vi "ZeitgrafBehandlung.vi"(6 "MaxArrayGröße":u16, 7 "error in":errorcluster, 8 "Temp-ArrayIn":dbl[](array[numeric]), 9 "Neue Temp":dbl, 10 "Neuer Zeitstempel":timestamp, 11 "Zeitstempel-ArrayIn":timestamp[](array[timestamp])) -> (0 "Temp-ArrayOut":dbl[](array[numeric]), 3 "Zeitstempel-ArrayOut":timestamp[](array[timestamp]), 4 "Temp-ZeitKurve":T1(graph), 5 "error out":errorcluster)   [LabVIEW 2024]
doc: "Dieses VI fügt eine Zeitstempel-Array und ein Werte-Array zusammen um Kurven anzuzeigen\nDabei werden die 2 Arrays zusätzlich verwaltet und auf eine Eingangsgröße beschränkt"
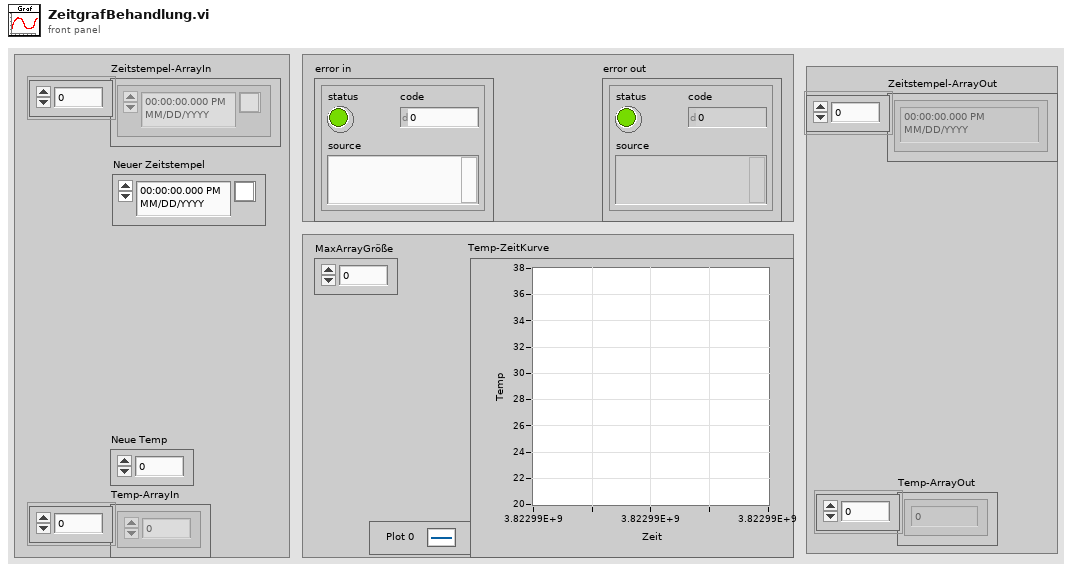
[diagram p1: front panel]
types:
  T1 = cluster{"Zeitstempel-ArrayIn ":timestamp[], "Temp-ArrayIn":dbl[]}
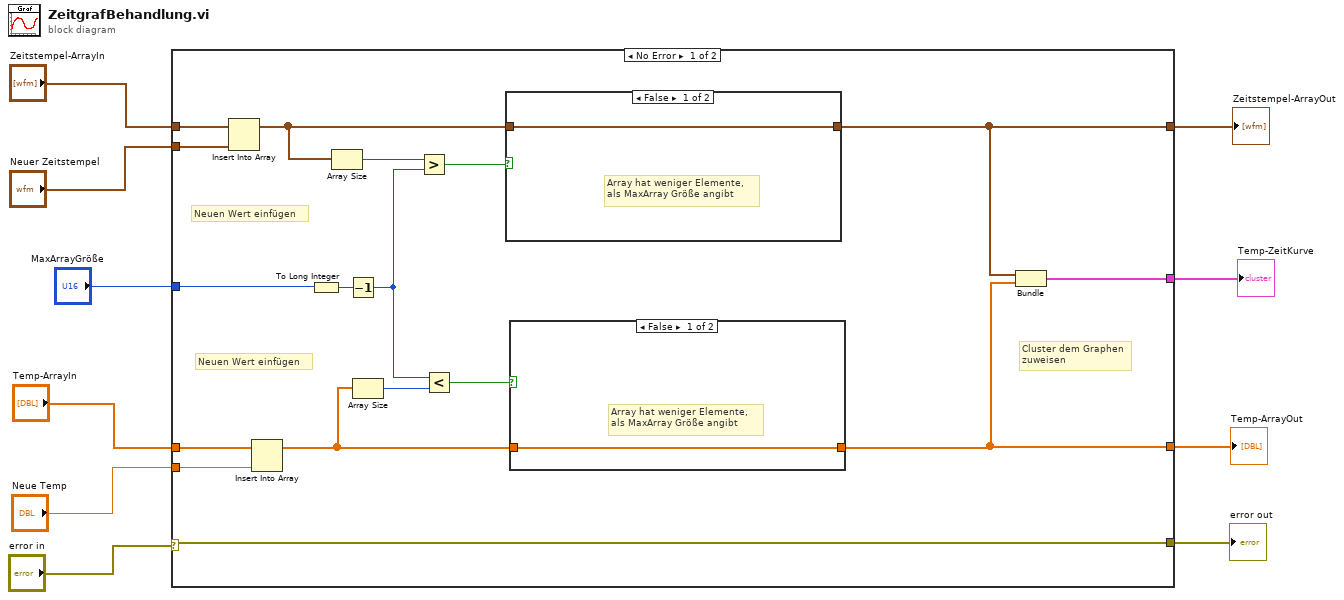
[diagram p0: block diagram]
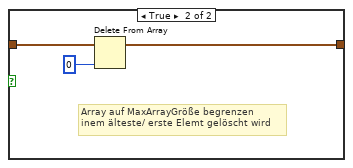
[diagram p2: hidden frame]
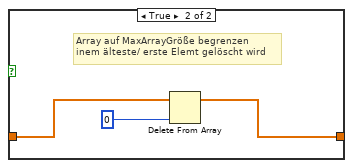
[diagram p3: hidden frame]
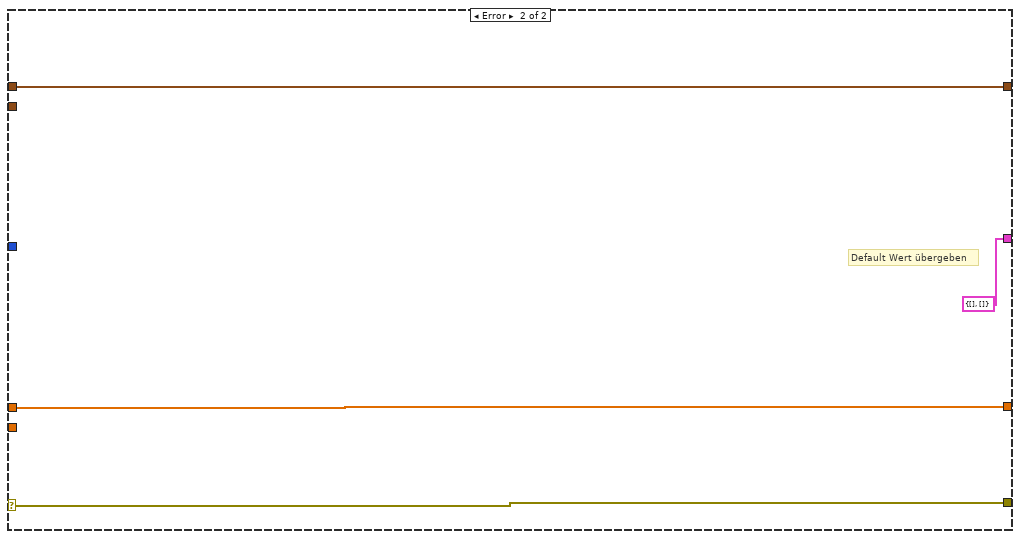
[diagram p4: hidden frame]
diagram:
  n1 = case shown="No Error" "error in" {
    selector: "error in" -> [w27 w38]
    tunnel: [w27 w38] -> w9
    tunnel: "Temp-ArrayIn" -> [w25 w39]
    tunnel: "Neue Temp" -> [w24 _]
    tunnel: "MaxArrayGröße" -> [w23 _]
    tunnel: "Zeitstempel-ArrayIn" -> [w22 w37]
    tunnel: "Neuer Zeitstempel" -> [w21 _]
    tunnel: [w15 w39] -> w3
    tunnel: [w19 T1 {"Zeitstempel-ArrayIn "=[], "Temp-ArrayIn"=[]}] -> w2
    tunnel: [w16 w37] -> w1
    frame No Error {
      # "Neuen Wert einfügen"
      # "Neuen Wert einfügen"
      # "Cluster dem Graphen zuweisen"
      n2 = Insert Into Array(array=w22, new element=w21) -> (w20:timestamp[])  [unwired: 1 in]
      n3 = Insert Into Array(array=w25, new element=w24) -> (w26:dbl[])  [unwired: 1 in]
      n4 = To Long Integer(number=w23) -> (32bit integer=w18:i32)
      n5 = Array Size(array=w20) -> (size(s)=w13:i32)
      n6 = Decrement(x=w18) -> (x-1=w12:i32)
      n7 = Array Size(array=w26) -> (size(s)=w11:i32)
      n8 = Greater?(x=w13, y=w12) -> (0:w14:bool)
      n9 = Less?(x=w12, y=w11) -> (x < y?=w17:bool)
      n10 = case shown="False" w14 {
        tunnel: w20 -> [w28 w31]
        tunnel: [w28 w29] -> w16
        frame False {
          # "Array hat weniger Elemente, \nals MaxArray Größe angibt"
        }
        frame True {
          # "Array auf MaxArrayGröße begrenzen\ninem älteste/ erste Elemt gelöscht wird"
          n11 = Delete From Array(array=w31, index=0) -> (array with subset deleted=w29:timestamp[])  [unwired: 1 in, 1 out]
        }
      }
      n12 = case shown="False" w17 {
        tunnel: w26 -> [w32 w35]
        tunnel: [w32 w33] -> w15
        frame False {
          # "Array hat weniger Elemente, \nals MaxArray Größe angibt"
        }
        frame True {
          # "Array auf MaxArrayGröße begrenzen\ninem älteste/ erste Elemt gelöscht wird"
          n13 = Delete From Array(array=w35, index=0) -> (array with subset deleted=w33:dbl[])  [unwired: 1 in, 1 out]
        }
      }
      n14 = Bundle("Zeitstempel-ArrayIn"=w16, "Temp-ArrayIn"=w15) -> (w19:T1)  [unwired: 1 in]
    }
    frame Error {
      # "Default Wert übergeben"
    }
  }
  "Zeitstempel-ArrayOut" <- w1
  "error out" <- w9
  "Temp-ArrayOut" <- w3
  "Temp-ZeitKurve" <- w2
